vi "LL_GET Service.vi"(8 "error in (no error)":errorcluster) -> (0 "error out":errorcluster, 1 "Call Result":T4, 3 "ListAllMyBucketsResult":T1)   [LabVIEW 2015, in "LV Interface for Amazon S3.lvlib"]
doc: "<b>Note</b>: This VI is no longer supported. Use the <b>Low-Level HTTP Request AWS v4</b> VI instead.\n\nThis implementation of the GET operation returns a list of all buckets owned by the authenticated sender of the request. Use this VI instead of the <B>List Buckets.vi</B> if you need more iformation than that returned by that VI."
uses:
  LV Interface for Amazon S3.lvlib
  Typedefs/AMZ_S3_Call Results.ctl
  Typedefs/AMZ_S3_API_ListAllMyBucketsResult.ctl
  Typedefs/AMZ_S3_API_Owner.ctl
  Typedefs/AMZ_S3_API_Bucket.ctl
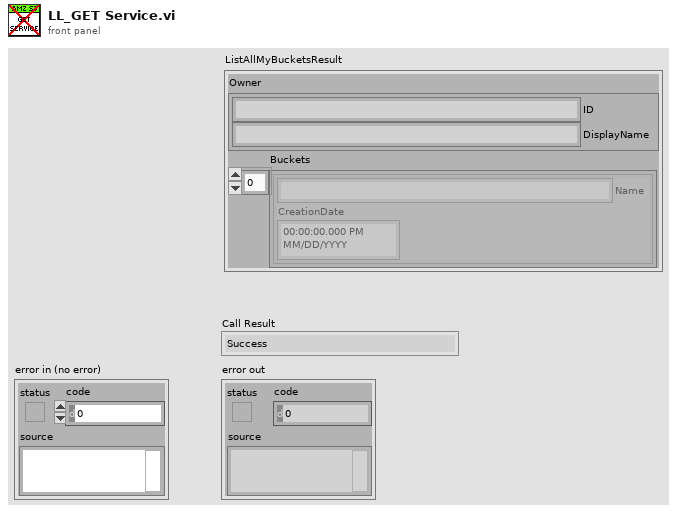
[diagram p1: front panel]
types:
  T1 = typedef "LV Interface for Amazon S3.lvlib/AMZ_S3_API_ListAllMyBucketsResult.ctl" = cluster{"Owner":T2, "Buckets":T3[]}
  T2 = typedef "LV Interface for Amazon S3.lvlib/AMZ_S3_API_Owner.ctl" = cluster{"ID":string, "DisplayName":string}
  T3 = typedef "LV Interface for Amazon S3.lvlib/AMZ_S3_API_Bucket.ctl" = cluster{"Name":string, "CreationDate":timestamp}
  T4 = typedef "LV Interface for Amazon S3.lvlib/AMZ_S3_Call Results.ctl" = enum16{"Success", "UndefinedError", "AccessDenied", "AccountProblem", "AmbiguousGrantByEmailAddress", "BadDigest", "BucketAlreadyExists", "BucketAlreadyOwnedByYou", "BucketNotEmpty", "CredentialsNotSupported", "CrossLocationLoggingProhibited", "EntityTooSmall", "EntityTooLarge", "ExpiredToken", "IllegalVersioningConfigurationException", "IncompleteBody", "IncorrectNumberOfFilesInPostRequest", "InlineDataTooLarge", "InternalError", "InvalidAccessKeyId", "InvalidAddressingHeader", "InvalidArgument", "InvalidBucketName", "InvalidDigest", "InvalidLocationConstraint", "InvalidPart", "InvalidPartOrder", "InvalidPayer", "InvalidPolicyDocument", "InvalidRange", "InvalidSecurity", "InvalidSOAPRequest", "InvalidStorageClass", "InvalidTargetBucketForLogging", "InvalidToken", "InvalidURI", "KeyTooLong", "MalformedACLError", "MalformedPOSTRequest", "MalformedXML", "MaxMessageLengthExceeded", "MaxPostPreDataLengthExceededError", "MetadataTooLarge", "MethodNotAllowed", "MissingAttachment", "MissingContentLength", "MissingRequestBodyError", "MissingSecurityElement", "MissingSecurityHeader", "NoLoggingStatusForKey", "NoSuchBucket", "NoSuchKey", "NoSuchUpload", "NoSuchVersion", "NotImplemented", "NotSignedUp", "OperationAborted", "PermanentRedirect", "PreconditionFailed", "Redirect", "RequestIsNotMultiPartContent", "RequestTimeout", "RequestTimeTooSkewed", "RequestTorrentOfBucketError", "SignatureDoesNotMatch", "SlowDown", "TemporaryRedirect", "TokenRefreshRequired", "TooManyBuckets", "UnexpectedContent", "UnresolvableGrantByEmailAddress", "UserKeyMustBeSpecified", "LabVIEWError"}
  T5 = cluster{"Value":string, "Time Stamp":timestamp}[]
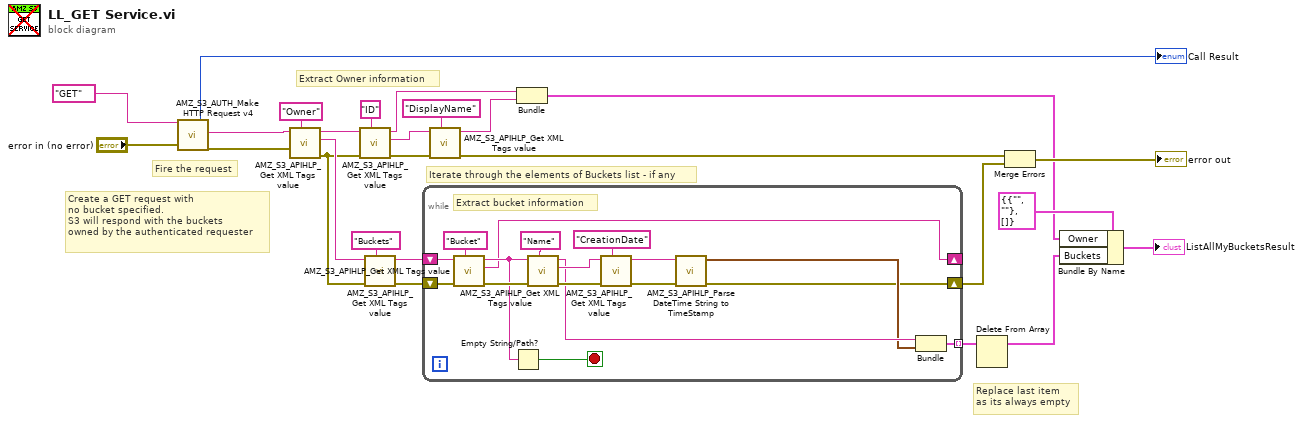
[diagram p0: block diagram]
diagram:
  # "Fire the request"
  # "Iterate through the elements of Buckets list - if any"
  # "Extract Owner information"
  # "Replace last item\nas its always empty"
  # "Create a GET request with\nno bucket specified.\nS3 will respond with the buckets\nowned by the authenticated requester"
  n1 = call "AMZ_S3_AUTH_Make HTTP Request v4.vi"("HTTP-Verb"="GET", "error in"="error in (no error)") -> ("Call Result"=→"Call Result":T4, "response body"=w2:string, "error out"=w3:errorcluster)  [unwired: 14 in, 1 out]
  n2 = call "AMZ_S3_APIHLP_Get XML Tags value.vi"("Tag name"="Owner", "error in (no error)"=w3, "XML String in"=w2) -> ("error out"=w17:errorcluster, "Remaining string"=w18:string, "Value"=w25:string)  [unwired: 6 in]
  n3 = call "AMZ_S3_APIHLP_Get XML Tags value.vi"("Tag name"="ID", "error in (no error)"=w17, "XML String in"=w25) -> ("error out"=w23:errorcluster, "Remaining string"=w22:string, "Value"=w19:string)  [unwired: 6 in]
  n4 = call "AMZ_S3_APIHLP_Get XML Tags value.vi"("Tag name"="Buckets", "error in (no error)"=w17, "XML String in"=w18) -> ("error out"=w15:errorcluster, "Value"=w14:string)  [unwired: 6 in, 1 out]
  n5 = while {
    shift-right: [w37] -> _
    shift-left: w14 -> [w42]
    tunnel: [w31] -> w13 mode=indexing
    shift-right: [w27] -> w11
    shift-left: w15 -> [w43]
    stop <- w41 stop-if-true
    # "Extract bucket information"
    n6 = call "AMZ_S3_APIHLP_Get XML Tags value.vi"("Tag name"="Bucket", "error in (no error)"=w43, "XML String in"=w42) -> ("error out"=w39:errorcluster, "Remaining string"=w37:string, "Value"=w38:string)  [unwired: 6 in]
    n7 = Empty String/Path?(string/path=w38) -> (empty?=w41:bool)
    n8 = call "AMZ_S3_APIHLP_Get XML Tags value.vi"("Tag name"="Name", "error in (no error)"=w39, "XML String in"=w38) -> ("error out"=w35:errorcluster, "Remaining string"=w34:string, "Value"=w32:string)  [unwired: 6 in]
    n9 = call "AMZ_S3_APIHLP_Get XML Tags value.vi"("Tag name"="CreationDate", "error in (no error)"=w35, "XML String in"=w34) -> ("error out"=w30:errorcluster, "Value"=w29:string)  [unwired: 6 in, 1 out]
    n10 = call "AMZ_S3_APIHLP_Parse DateTime String to TimeStamp.vi"("error in (no error)"=w30, "DateTime String"=w29) -> ("error out"=w27:errorcluster, "Time Stamp"=w28:timestamp)  [unwired: 8 in]
    n11 = Bundle("Value"=w32, "Time Stamp"=w28) -> (w31:cluster{"Value":string, "Time Stamp":timestamp})  [unwired: 1 in]
  }
  n12 = call "AMZ_S3_APIHLP_Get XML Tags value.vi"("Tag name"="DisplayName", "error in (no error)"=w23, "XML String in"=w22) -> ("error out"=w12:errorcluster, "Value"=w20:string)  [unwired: 6 in, 1 out]
  n13 = Bundle("Value"=w19, "Value"=w20) -> (w7:cluster{"Value":string, "Value":string})  [unwired: 1 in]
  n14 = Delete From Array(array=w13) -> (array with subset deleted=w8:T5)  [unwired: 2 in, 1 out]
  n15 = Merge Errors(w12, w11) -> (→"error out":errorcluster)
  n16 = Bundle By Name(cluster=T1 {"Owner"={"ID"="", "DisplayName"=""}, "Buckets"=[]} ("ListAllMyBucketsResult"), "Owner"=w7, "Buckets"=w8) -> (→"ListAllMyBucketsResult":T1)
